vi "Write Faulty Message (TCP).vi"(5 "message length [bytes] (-1: calculate)":i64=-1, 6 "options":T1={"ignore timeout error"=TRUE, "timeout ms (1000)"=1000}, 7 "meta data index [bytes] (-1: lookup)":i32=-1, 8 "error in":errorcluster, 9 "data (\"\")":string, 10 "name (\"\")":string, 11 "connection info in":T2) -> (0 "error out":errorcluster, 3 "connection info out":T2)   [LabVIEW 2013]
doc: "This VI writes <b>an intentionally faulty</b> package of data to a remote computer. It prepends a <b>configurable</b> meta data ID number to each packet. This is useful when developing unit tests.\n\nIf <b>meta data index</b> and <b>message length</b> are left unwired, this VI sends a valid message in the same way as Write Message (TCP).vi."
uses:
  vi.lib/NI/STM/TCP/TCP Connection Info.ctl
  vi.lib/NI/STM/SubVIs/MetaDataElement.ctl
  vi.lib/NI/STM/TCP/TCP Write Options.ctl
  vi.lib/NI/STM/NI STM.lvlib
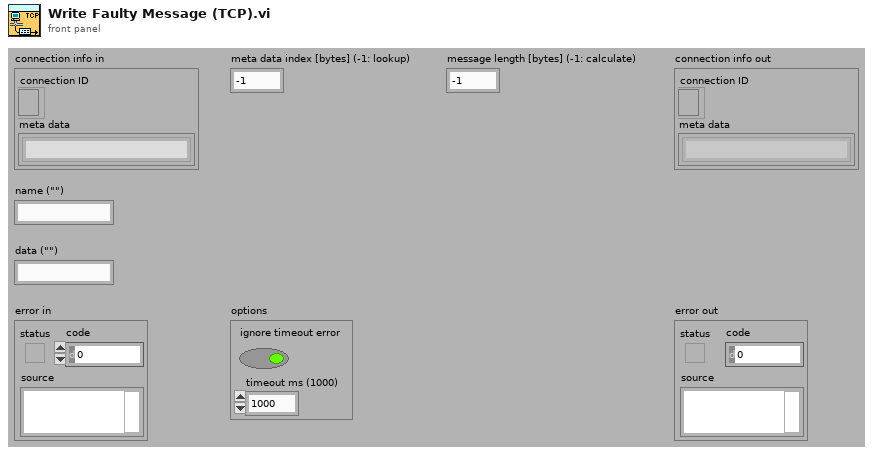
[diagram p1: front panel]
types:
  T1 = typedef "NI STM.lvlib/TCP Write Options.ctl" = cluster{"ignore timeout error":bool, "timeout ms (1000)":i32}
  T2 = typedef "NI STM.lvlib/TCP Connection Info.ctl" = cluster{"connection ID":refnum<k5>, "meta data":T3[]}
  T3 = typedef "NI STM.lvlib/MetaDataElement.ctl" = string
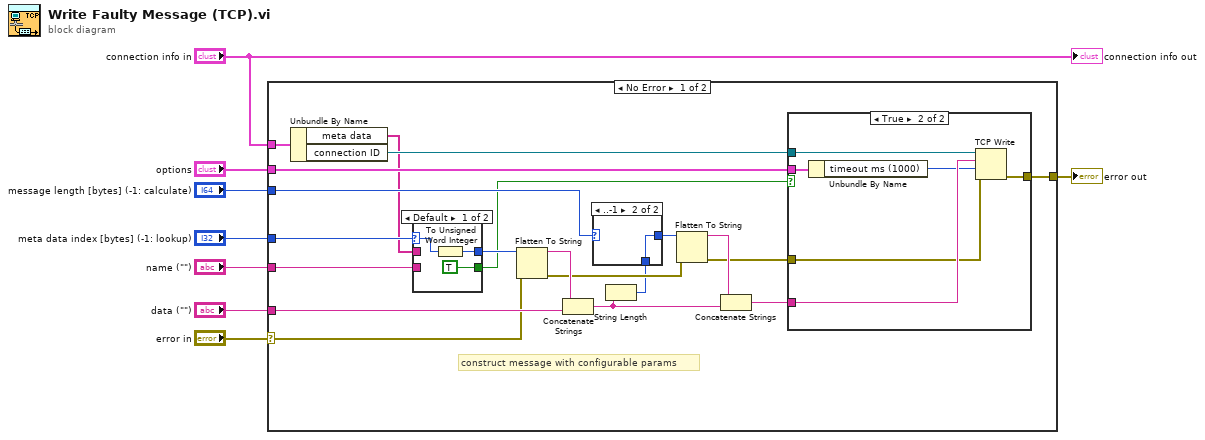
[diagram p0: block diagram]
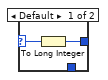
[diagram p2: hidden frame]
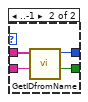
[diagram p3: hidden frame]
diagram:
  n1 = case shown="No Error" "error in" {
    selector: "error in" -> [w12 w46]
    tunnel: "connection info in" -> [w26 _]
    tunnel: [w28 w46] -> w8
    tunnel: "name (\"\")" -> [w16 _]
    tunnel: "data (\"\")" -> [w21 _]
    tunnel: "options" -> [w25 _]
    tunnel: "meta data index [bytes] (-1: lookup)" -> [w24 _]
    tunnel: "message length [bytes] (-1: calculate)" -> [w18 _]
    frame No Error {
      # "construct message with configurable params"
      n2 = Unbundle By Name(w26) -> ("meta data"=w17:T3[], "connection ID"=w27:refnum<k5>)
      n3 = case shown="Default" w24 {
        selector: w24 -> [w34 _]
        tunnel: [w33 w38] -> w22
        tunnel: [TRUE ("found?") w37] -> w11
        tunnel: w17 -> [_ w36]
        tunnel: w16 -> [_ w35]
        frame Default {
          n4 = To Unsigned Word Integer(number=w34) -> (unsigned 16bit integer=w33:u16)
        }
        frame ..-1 {
          n5 = call "GetIDfromName.vi"("name"=w35, "meta data"=w36) -> ("found?"=w37:bool, "meta ID"=w38:u16)  [unwired: 8 out]
        }
      }
      n6 = Flatten To String(anything=w22, error in (no error)=w12) -> (data string=w23:string, error out=w19:errorcluster)  [unwired: 3 out]
      n7 = Concatenate Strings(w23, w21) -> (w14:string)
      n8 = String Length(string=w14) -> (length=w13:i32)
      n9 = case shown="..-1" w18 {
        selector: w18 -> [w30 _]
        tunnel: [w29 w31] -> w20
        tunnel: w13 -> [_ w31]
        frame Default {
          n10 = To Long Integer(number=w30) -> (32bit integer=w29:i32)
        }
        frame ..-1 {
        }
      }
      n11 = Flatten To String(anything=w20, error in (no error)=w19) -> (data string=w15:string, error out=w10:errorcluster)  [unwired: 3 out]
      n12 = Concatenate Strings(w15, w14) -> (w9:string)
      n13 = case shown="True" w11 {
        tunnel: w27 -> [_ w45]
        tunnel: w10 -> [w39 w42]
        tunnel: [w39 w44] -> w28
        tunnel: w9 -> [_ w43]
        tunnel: w25 -> [_ w40]
        frame False {
        }
        frame True {
          n14 = Unbundle By Name(w40) -> ("timeout ms (1000)"=w41:i32)
          n15 = TCP Write(connection ID=w45, data in=w43, error in (no error)=w42, 9:w41) -> (error out=w44:errorcluster)  [unwired: 2 out]
        }
      }
    }
    frame Error {
    }
  }
  "error out" <- w8
  "connection info out" <- "connection info in"
